vi "控制命令.vi"(8 "Error in":errorcluster caption="Error in (no error)", 11 "参数":T1={"站号"=1, "量程切换"=enum."AUTO", "控制命令"=enum."启动测量", "模式设置"=enum."待机", "测量间隔"=0} {"站号" items=["总磷"=1, "氨氮"=3]}) -> (0 "error out":errorcluster)   [LabVIEW 2016, in "斯坦道氨氮.lvlib"]
uses:
  <vilib>/Plasmionique/MB Master/MB_Master/MB_Master.lvclass
  <vilib>/Plasmionique/MB Master/MB Master.lvlib
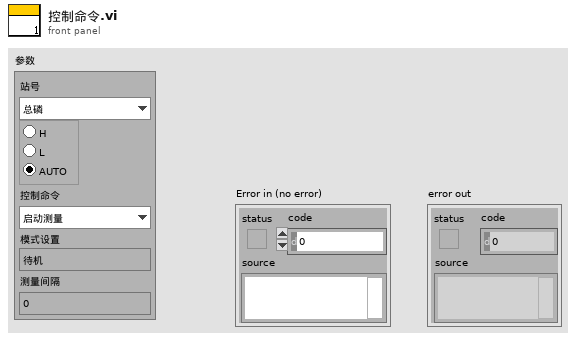
[diagram p1: front panel]
types:
  T1 = cluster{"站号":u16, "量程切换":enum32{"H", "L", "AUTO"}, "控制命令":enum16{"启动测量", "标样核查", "零点核查", "跨度核查", "空白测试", "平行样测试", "加标回收", "空白校准", "标样校准", "初始化（清洗）", "停止测试", "仪器重启", "校时", "模式设置", "测量间隔设置", ""}, "模式设置":enum16{"待机", "连续模式", "周期模式", "定点模式", "受控模式", "手动模式"}, "测量间隔":u16}
  T2 = enum16{"启动测量", "标样核查", "零点核查", "跨度核查", "空白测试", "平行样测试", "加标回收", "空白校准", "标样校准", "初始化（清洗）", "停止测试", "仪器重启", "校时", "模式设置", "测量间隔设置", ""}
  T3 = enum16{"待机", "连续模式", "周期模式", "定点模式", "受控模式", "手动模式"}
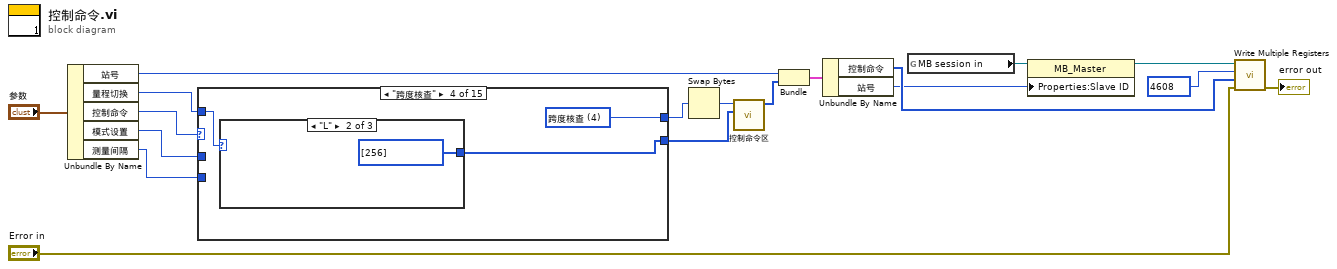
[diagram p0: block diagram]
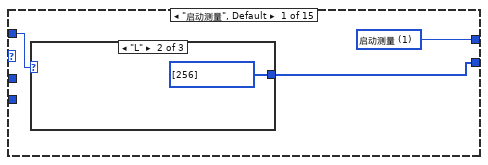
[diagram p2: hidden frame]
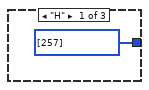
[diagram p3: hidden frame]
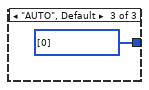
[diagram p4: hidden frame]
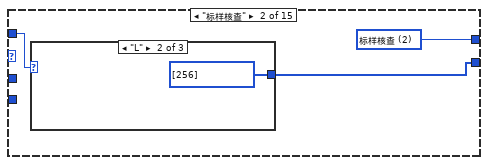
[diagram p5: hidden frame]
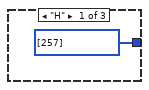
[diagram p6: hidden frame]
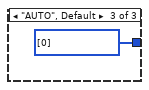
[diagram p7: hidden frame]
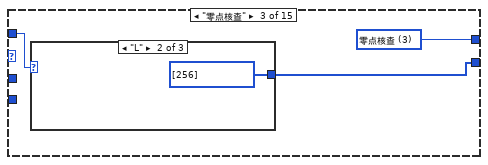
[diagram p8: hidden frame]
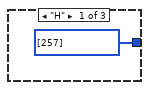
[diagram p9: hidden frame]
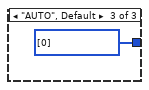
[diagram p10: hidden frame]
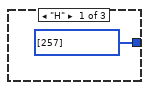
[diagram p11: hidden frame]
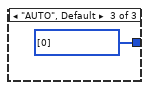
[diagram p12: hidden frame]
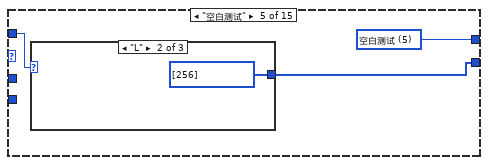
[diagram p13: hidden frame]
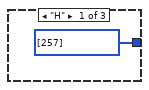
[diagram p14: hidden frame]
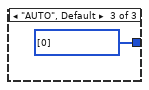
[diagram p15: hidden frame]
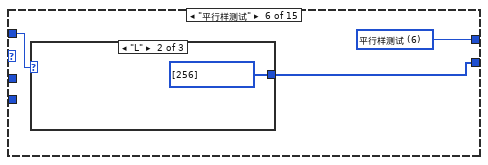
[diagram p16: hidden frame]
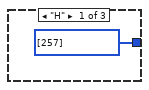
[diagram p17: hidden frame]
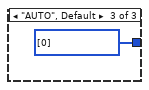
[diagram p18: hidden frame]
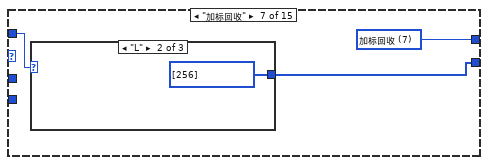
[diagram p19: hidden frame]
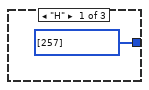
[diagram p20: hidden frame]
diagram:
  n1 = Unbundle By Name("参数") -> ("站号"=w17:u16, "量程切换"=w16:enum32{"H", "L", "AUTO"}, "控制命令"=w15:T2, "模式设置"=w13:T3, "测量间隔"=w14:u16)
  n2 = case shown="\"跨度核查\"" w15 {
    tunnel: [w19 w25 w31 w37 w43 w49 w55 w61 w67 i32[] [] i32[] [] i32[] [] w79 w85 w95] -> w10
    tunnel: w16 -> [w21 w27 w33 w39 w45 w51 w57 w63 w69 _ _ _ _ _ _]
    tunnel: [w20 w26 w32 w38 w44 w50 w56 w62 w68 w73 w75 w77 w80 w87 w97] -> w9
    tunnel: w14 -> [_ _ _ _ _ _ _ _ _ _ _ _ _ _ w94]
    tunnel: w13 -> [_ _ _ _ _ _ _ _ _ _ _ _ _ w84 _]
    frame "启动测量", Default {
      w20 = u16 1 items=["启动测量"=1, "标样核查"=2, "零点核查"=3, "跨度核查"=4, "空白测试"=5, "平行样测试"=6, "加标回收"=7, "空白校准"=8, "标样校准"=9, "初始化（清洗）"=10, "停止测试"=11, "仪器重启"=12, "校时"=13, "模式设置"=14, "测量间隔设置"=15] ("控制命令")
      n3 = case shown="\"L\"" w21 {
        tunnel: [i32[] [257] i32[] [256] i32[] [0]] -> w19
        frame "H" {
        }
        frame "L" {
        }
        frame "AUTO", Default {
        }
      }
    }
    frame "标样核查" {
      w26 = u16 2 items=["启动测量"=1, "标样核查"=2, "零点核查"=3, "跨度核查"=4, "空白测试"=5, "平行样测试"=6, "加标回收"=7, "空白校准"=8, "标样校准"=9, "初始化（清洗）"=10, "停止测试"=11, "仪器重启"=12, "校时"=13, "模式设置"=14, "测量间隔设置"=15] ("控制命令")
      n4 = case shown="\"L\"" w27 {
        tunnel: [i32[] [257] i32[] [256] i32[] [0]] -> w25
        frame "H" {
        }
        frame "L" {
        }
        frame "AUTO", Default {
        }
      }
    }
    frame "零点核查" {
      w32 = u16 3 items=["启动测量"=1, "标样核查"=2, "零点核查"=3, "跨度核查"=4, "空白测试"=5, "平行样测试"=6, "加标回收"=7, "空白校准"=8, "标样校准"=9, "初始化（清洗）"=10, "停止测试"=11, "仪器重启"=12, "校时"=13, "模式设置"=14, "测量间隔设置"=15] ("控制命令")
      n5 = case shown="\"L\"" w33 {
        tunnel: [i32[] [257] i32[] [256] i32[] [0]] -> w31
        frame "H" {
        }
        frame "L" {
        }
        frame "AUTO", Default {
        }
      }
    }
    frame "跨度核查" {
      w38 = u16 4 items=["启动测量"=1, "标样核查"=2, "零点核查"=3, "跨度核查"=4, "空白测试"=5, "平行样测试"=6, "加标回收"=7, "空白校准"=8, "标样校准"=9, "初始化（清洗）"=10, "停止测试"=11, "仪器重启"=12, "校时"=13, "模式设置"=14, "测量间隔设置"=15] ("控制命令")
      n6 = case shown="\"L\"" w39 {
        tunnel: [i32[] [257] i32[] [256] i32[] [0]] -> w37
        frame "H" {
        }
        frame "L" {
        }
        frame "AUTO", Default {
        }
      }
    }
    frame "空白测试" {
      w44 = u16 5 items=["启动测量"=1, "标样核查"=2, "零点核查"=3, "跨度核查"=4, "空白测试"=5, "平行样测试"=6, "加标回收"=7, "空白校准"=8, "标样校准"=9, "初始化（清洗）"=10, "停止测试"=11, "仪器重启"=12, "校时"=13, "模式设置"=14, "测量间隔设置"=15] ("控制命令")
      n7 = case shown="\"L\"" w45 {
        tunnel: [i32[] [257] i32[] [256] i32[] [0]] -> w43
        frame "H" {
        }
        frame "L" {
        }
        frame "AUTO", Default {
        }
      }
    }
    frame "平行样测试" {
      w50 = u16 6 items=["启动测量"=1, "标样核查"=2, "零点核查"=3, "跨度核查"=4, "空白测试"=5, "平行样测试"=6, "加标回收"=7, "空白校准"=8, "标样校准"=9, "初始化（清洗）"=10, "停止测试"=11, "仪器重启"=12, "校时"=13, "模式设置"=14, "测量间隔设置"=15] ("控制命令")
      n8 = case shown="\"L\"" w51 {
        tunnel: [i32[] [257] i32[] [256] i32[] [0]] -> w49
        frame "H" {
        }
        frame "L" {
        }
        frame "AUTO", Default {
        }
      }
    }
    frame "加标回收" {
      w56 = u16 7 items=["启动测量"=1, "标样核查"=2, "零点核查"=3, "跨度核查"=4, "空白测试"=5, "平行样测试"=6, "加标回收"=7, "空白校准"=8, "标样校准"=9, "初始化（清洗）"=10, "停止测试"=11, "仪器重启"=12, "校时"=13, "模式设置"=14, "测量间隔设置"=15] ("控制命令")
      n9 = case shown="\"L\"" w57 {
        tunnel: [i32[] [257] i32[] [256] i32[] [0]] -> w55
        frame "H" {
        }
        frame "L" {
        }
        frame "AUTO", Default {
        }
      }
    }
    frame "空白校准" {
      w62 = u16 8 items=["启动测量"=1, "标样核查"=2, "零点核查"=3, "跨度核查"=4, "空白测试"=5, "平行样测试"=6, "加标回收"=7, "空白校准"=8, "标样校准"=9, "初始化（清洗）"=10, "停止测试"=11, "仪器重启"=12, "校时"=13, "模式设置"=14, "测量间隔设置"=15] ("控制命令")
      n10 = case shown="\"L\"" w63 {
        tunnel: [i32[] [257] i32[] [256] i32[] [0]] -> w61
        frame "H" {
        }
        frame "L" {
        }
        frame "AUTO", Default {
        }
      }
    }
    frame "标样校准" {
      w68 = u16 9 items=["启动测量"=1, "标样核查"=2, "零点核查"=3, "跨度核查"=4, "空白测试"=5, "平行样测试"=6, "加标回收"=7, "空白校准"=8, "标样校准"=9, "初始化（清洗）"=10, "停止测试"=11, "仪器重启"=12, "校时"=13, "模式设置"=14, "测量间隔设置"=15] ("控制命令")
      n11 = case shown="\"L\"" w69 {
        tunnel: [i32[] [257] i32[] [256] i32[] [0]] -> w67
        frame "H" {
        }
        frame "L" {
        }
        frame "AUTO", Default {
        }
      }
    }
    frame "初始化（清洗）" {
      w73 = u16 10 items=["启动测量"=1, "标样核查"=2, "零点核查"=3, "跨度核查"=4, "空白测试"=5, "平行样测试"=6, "加标回收"=7, "空白校准"=8, "标样校准"=9, "初始化（清洗）"=10, "停止测试"=11, "仪器重启"=12, "校时"=13, "模式设置"=14, "测量间隔设置"=15] ("控制命令")
    }
    frame "停止测试" {
      w75 = u16 11 items=["启动测量"=1, "标样核查"=2, "零点核查"=3, "跨度核查"=4, "空白测试"=5, "平行样测试"=6, "加标回收"=7, "空白校准"=8, "标样校准"=9, "初始化（清洗）"=10, "停止测试"=11, "仪器重启"=12, "校时"=13, "模式设置"=14, "测量间隔设置"=15] ("控制命令")
    }
    frame "仪器重启" {
      w77 = u16 12 items=["启动测量"=1, "标样核查"=2, "零点核查"=3, "跨度核查"=4, "空白测试"=5, "平行样测试"=6, "加标回收"=7, "空白校准"=8, "标样校准"=9, "初始化（清洗）"=10, "停止测试"=11, "仪器重启"=12, "校时"=13, "模式设置"=14, "测量间隔设置"=15] ("控制命令")
    }
    frame "校时" {
      w80 = u16 13 items=["启动测量"=1, "标样核查"=2, "零点核查"=3, "跨度核查"=4, "空白测试"=5, "平行样测试"=6, "加标回收"=7, "空白校准"=8, "标样校准"=9, "初始化（清洗）"=10, "停止测试"=11, "仪器重启"=12, "校时"=13, "模式设置"=14, "测量间隔设置"=15] ("控制命令")
      n12 = Get Date/Time In Seconds() -> (seconds since 1Jan1904=w83:timestamp)
      n13 = Insert Into Array(array=timestamp[] [] ("数组"), new element=w83) -> (w81:timestamp[])  [unwired: 1 in]
      n14 = call "DateToHex.vi"("DATE"=w81) -> ("数组"=w79:u16[])  [unwired: 10 in]
    }
    frame "模式设置" {
      w87 = u16 14 items=["启动测量"=1, "标样核查"=2, "零点核查"=3, "跨度核查"=4, "空白测试"=5, "平行样测试"=6, "加标回收"=7, "空白校准"=8, "标样校准"=9, "初始化（清洗）"=10, "停止测试"=11, "仪器重启"=12, "校时"=13, "模式设置"=14, "测量间隔设置"=15] ("控制命令")
      n15 = case shown="\"手动模式\"" w84 {
        tunnel: [i32[] [0] i32[] [1] i32[] [2] i32[] [3] i32[] [4] i32[] [5]] -> w86
        frame "待机", Default {
        }
        frame "连续模式" {
        }
        frame "周期模式" {
        }
        frame "定点模式" {
        }
        frame "受控模式" {
        }
        frame "手动模式" {
        }
      }
      n16 = call "HexToWord.vi"("数组"=w86) -> ("WORD"=w85:u16[])  [unwired: 10 in]
    }
    frame "测量间隔设置" {
      w97 = u16 15 items=["启动测量"=1, "标样核查"=2, "零点核查"=3, "跨度核查"=4, "空白测试"=5, "平行样测试"=6, "加标回收"=7, "空白校准"=8, "标样校准"=9, "初始化（清洗）"=10, "停止测试"=11, "仪器重启"=12, "校时"=13, "模式设置"=14, "测量间隔设置"=15] ("控制命令")
      n17 = Replace Array Subset(array=i32[] [0], new element=w94) -> (w96:i32[])  [unwired: 1 in]
      n18 = call "HexToWord.vi"("数组"=w96) -> ("WORD"=w95:u16[])  [unwired: 10 in]
    }
  }
  n19 = Swap Bytes(anything=w9) -> (byte swapped=w8:u16)
  n20 = call "控制命令区.vi"("控制命令参数"=w10, "控制命令"=w8) -> ("控制命令"=w11:u16[])  [unwired: 9 in]
  n21 = Bundle("站号"=w17, "控制命令"=w11) -> (w12:cluster{"站号":u16, "控制命令":u16[]})  [unwired: 1 in]
  n22 = Unbundle By Name(w12) -> ("控制命令"=w5:u16[], "站号"=w3:u16)
  n23 = global read "VAR总磷总氮全局变量.vi" "MB session in"() -> (w7:refnum<class "MB_Master.lvclass">)
  n24 = property class="MB_Master"(reference=w7, "Properties:Slave ID"=w3) -> (reference out=w4:refnum<class "MB_Master.lvclass">)  [unwired: 1 in, 1 out]
  n25 = call <vilib>:"Write Multiple Registers.vi"("error in (no error)"="Error in", "values"=w5, "starting address"=u16 4608, "MB session in"=w4) -> ("error out"=→"error out":errorcluster)  [unwired: 6 in, 1 out]
